vi "Set Print Speeds.vi"(8 "error in (no error)":errorcluster, 9 "Enum":enum16{"Mixer", "Screw"}(ring)=enum."Screw", 10 "Speed":i32, 11 "Feeder Actor.lvlib:Feeder.lvclass":refnum<class "Feeder.lvclass">) -> (0 "error out":errorcluster, 3 "Feeder Actor.lvlib:Feeder.lvclass 2":refnum<class "Feeder.lvclass">)   [LabVIEW 2018, in "Feeder Actor.lvlib" / "Feeder.lvclass"]
uses:
  Feeder.lvclass
  Feeder.lvclass/Feeder.ctl
  Screw Messages/Set Screw Printing Speed Msg/Set Screw Printing Speed Msg.lvclass
  Mixer Messages/Set Mixer Printing Speed Msg/Set Mixer Printing Speed Msg.lvclass
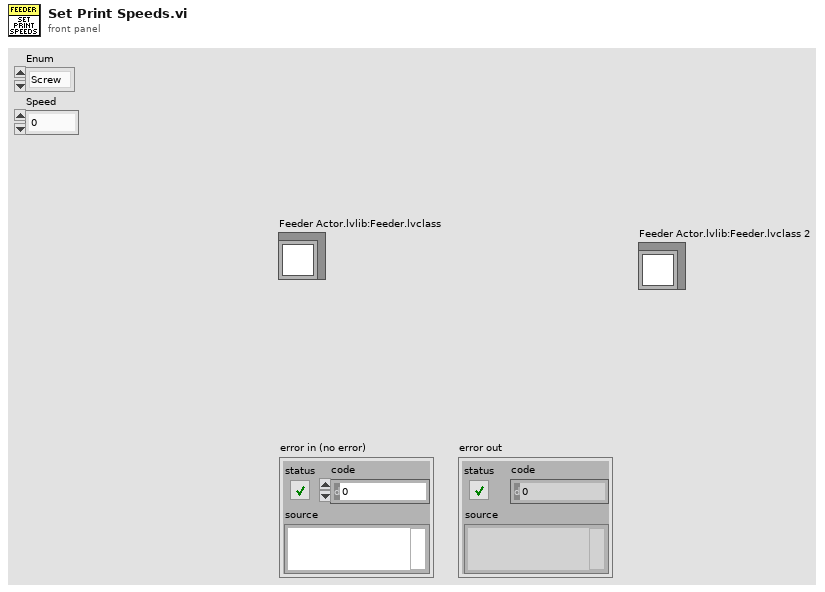
[diagram p1: front panel]
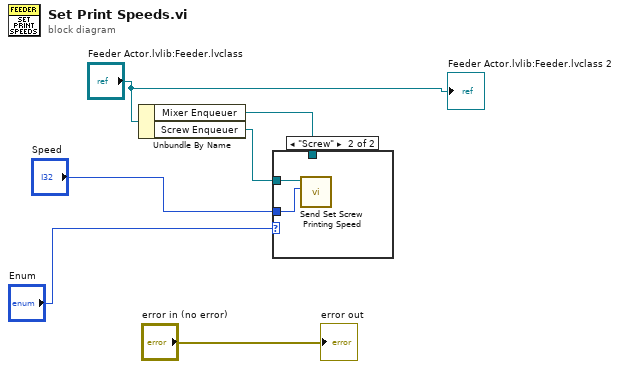
[diagram p0: block diagram]
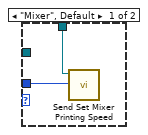
[diagram p2: hidden frame]
diagram:
  n1 = Unbundle By Name("Feeder Actor.lvlib:Feeder.lvclass") -> ("Mixer Enqueuer"=w2:refnum<class "Message Enqueuer.lvclass">, "Screw Enqueuer"=w6:refnum<class "Message Enqueuer.lvclass">)
  n2 = case shown="\"Screw\"" "Enum" {
    tunnel: w6 -> [_ w10]
    tunnel: w2 -> [w8 _]
    tunnel: "Speed" -> [w7 w9]
    frame "Mixer", Default {
      n3 = call "Send Set Mixer Printing Speed.vi"("Print Speed"=w7, "Message Enqueuer in"=w8) -> ()  [unwired: 8 in, 2 out]
    }
    frame "Screw" {
      n4 = call "Send Set Screw Printing Speed.vi"("Print Speed"=w9, "Message Enqueuer in"=w10) -> ()  [unwired: 8 in, 2 out]
    }
  }
  "Feeder Actor.lvlib:Feeder.lvclass 2" <- "Feeder Actor.lvlib:Feeder.lvclass"
  "error out" <- "error in (no error)"
